vi "Scale Picture to Centre Image.vi"(7 "Erase First? (Default: True)":bool=TRUE, 8 "error in (no error)":errorcluster, 10 "Image Size":T2, 11 "Picture in":refnum<vi>) -> (0 "error out":errorcluster, 1 "Zoom Factor Set":dbl, 3 "Draw Image to Picture Offset":T1)   [LabVIEW 2020, in "image.lvlib"]
doc: "Set the Zoom Factor of a LabVIEW Picture Control and Compute the Picture Offset to pass to \"Draw Image.vi\" so that the Image will fill the Picture Control and be vertically and horizontally centred."
uses:
  image.lvlib
  common/Image Size (Integer).ctl
  Image Draw Offset.ctl
  common/common.lvlib
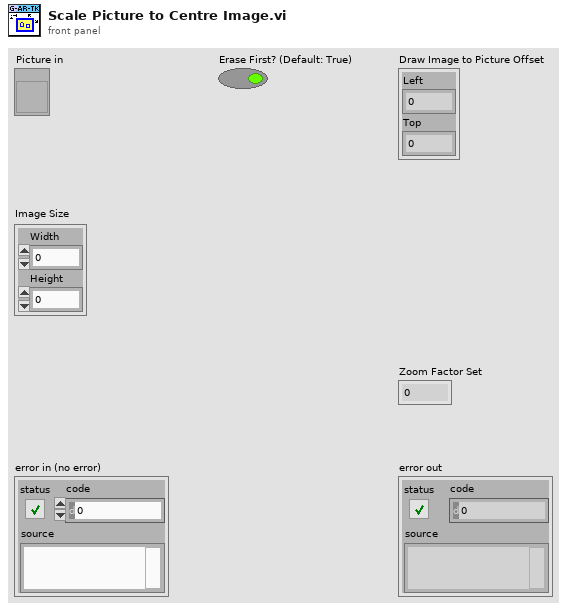
[diagram p1: front panel]
types:
  T1 = typedef "image.lvlib/Image Draw Offset.ctl" = cluster{"Left":i16, "Top":i16}
  T2 = typedef "common.lvlib/Image Size (Integer).ctl" = cluster{"Width":u16, "Height":u16}
  T3 = typedef "LVBoundsTypeDef.ctl" = cluster{"Width":u32, "Height":u32}
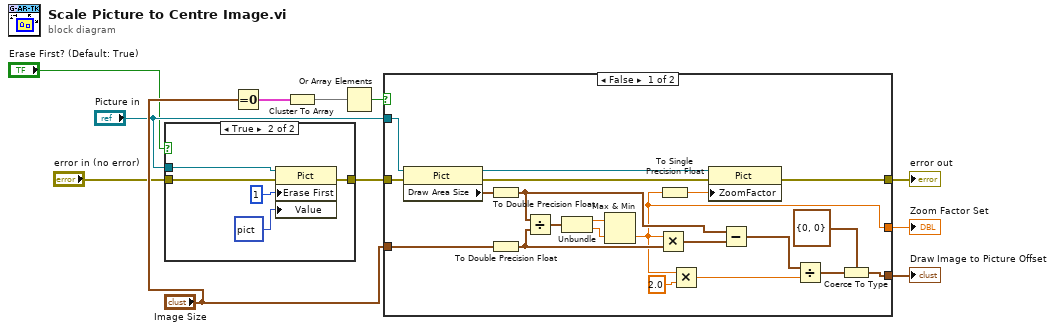
[diagram p0: block diagram]
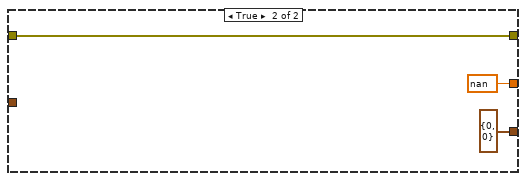
[diagram p3: hidden frame]
diagram:
  n1 = case shown="True" "Erase First? (Default: True)" {
    tunnel: [w12 w17] -> w3
    tunnel: "Picture in" -> [_ w16]
    tunnel: "error in (no error)" -> [w12 w15]
    frame False {
    }
    frame True {
      n2 = property on="Property Node" class="Pict"(reference=w16, error in=w15, "Erase First"=u8 1, "Value"=picture data[5B] ("empty picture")) -> (error out=w17:errorcluster)  [unwired: 1 out]
    }
  }
  n3 = Equal To 0?(x="Image Size") -> (x = 0?=w9:cluster{"Width":bool, "Height":bool})
  n4 = Cluster To Array(cluster=w9) -> (array=w8:bool[])
  n5 = Or Array Elements(Boolean array=w8) -> (logical OR=w6:bool)
  n6 = case shown="False" w6 {
    tunnel: "Picture in" -> [w18 _]
    tunnel: w3 -> [w19 w41]
    tunnel: [w35 T1 {"Left"=0, "Top"=0} ("Image Draw Offset (Default 0,0)")] -> w11
    tunnel: "Image Size" -> [w34 _]
    tunnel: [w33 w41] -> w7
    tunnel: [w21 nan] -> w5
    frame False {
      n7 = property on="Property Node" class="Pict"(reference=w18, error in=w19) -> (reference out=w30:refnum<vi>, error out=w31:errorcluster, "Draw Area Size"=w32:T3)
      n8 = To Double Precision Float(number=w32) -> (double precision float=w26:cluster{"Width":dbl, "Height":dbl})
      n9 = To Double Precision Float(number=w34) -> (double precision float=w27:cluster{"Width":dbl, "Height":dbl})
      n10 = Divide(x=w26, y=w27) -> (x/y=w38:cluster{"Width":dbl, "Height":dbl})
      n11 = Unbundle(w38) -> ("Width"=w28:dbl, "Height"=w29:dbl)
      n12 = Max & Min(x=w28, y=w29) -> (min(x,y)=w21:dbl)  [unwired: 1 out]
      n13 = Multiply(x=w21, y=w27) -> (x*y=w25:cluster{"Width":dbl, "Height":dbl})
      n14 = To Single Precision Float(number=w21) -> (single precision float=w37:sgl)
      n15 = Multiply(x=w21, y=2.0) -> (x*y=w22:dbl)
      n16 = property on="Property Node" class="Pict"(reference=w30, error in=w31, "ZoomFactor"=w37) -> (error out=w33:errorcluster)  [unwired: 1 out]
      n17 = Subtract(x=w26, y=w25) -> (x-y=w24:cluster{"Width":dbl, "Height":dbl})
      n18 = Divide(x=w24, y=w22) -> (x/y=w20:cluster{"Width":dbl, "Height":dbl})
      n19 = Coerce To Type(0:w20, 1:T1 {"Left"=0, "Top"=0} ("Image Draw Offset (Default 0,0)")) -> (2:w35:T1)
    }
    frame True {
    }
  }
  "Draw Image to Picture Offset" <- w11
  "error out" <- w7
  "Zoom Factor Set" <- w5
